vi "Get Photons.vi"(10 "in range":bool=TRUE, 11 "mark valid location":bool) -> (3 "read output":T1)   [LabVIEW 2010]
uses:
  common_typedefs/channels_cluster.ctl
  <vilib>/rvi/DataTransferAndStorage/Container/XNode/niFpgaContainer.xnode
  <vilib>/rvi/FIFO/Fifo_Resource/nirvififoEmulationSetSize.vi
  <vilib>/rvi/DataTransferAndStorage/Container/Common/niFpgaContainerGetUniqueNameForEmu.vi
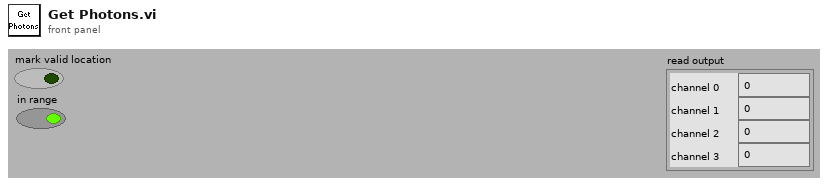
[diagram p1: front panel]
types:
  T1 = typedef "channels_cluster.ctl" = cluster{"channel 0":u32, "channel 1":u32, "channel 2":u32, "channel 3":u32}
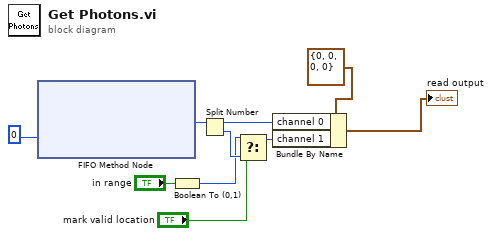
[diagram p0: block diagram]
diagram:
  n1 = xnode ("FIFO Method Node")("Timeout"=0) -> ("Element"=w8:u64)  [unwired: 1 in, 2 out]
  n2 = Boolean To (0,1)(Boolean="in range") -> (0, 1=w2:i16)
  n3 = Split Number(x=w8) -> (hi(x)=w7:u32, lo(x)=w4:u32)
  n4 = Select(t=w2, s="mark valid location", f=w4) -> (s? t:f=w5:u32)
  n5 = Bundle By Name(cluster=T1 {"channel 0"=0, "channel 1"=0, "channel 2"=0, "channel 3"=0} ("read output"), "channel 0"=w7, "channel 1"=w5) -> (→"read output":T1)
